vi "Write Properties.vi"(10 "Properties":refnum<class "Properties.lvclass">, 11 "Leaf.Properties in":refnum<class "Leaf.Properties.lvclass">) -> (3 "Leaf.Properties out":refnum<class "Leaf.Properties.lvclass">)   [LabVIEW 2021, in "Banana.Caraya.lvlib" / "Leaf.Properties.lvclass"]
uses:
  Leaf.Properties.lvclass
  Leaf.Properties.lvclass/Leaf.Properties.ctl
  <vilib>/addons/_JKI Toolkits/Caraya/classes/Properties/Properties.lvclass
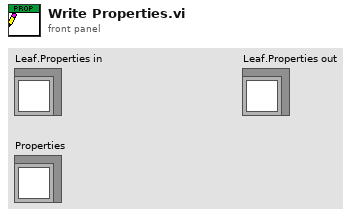
[diagram p1: front panel]
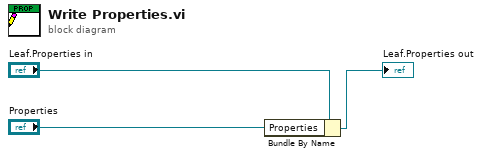
[diagram p0: block diagram]
diagram:
  n1 = Bundle By Name(cluster="Leaf.Properties in", "Properties"="Properties") -> (→"Leaf.Properties out":refnum<class "Leaf.Properties.lvclass">)
